vi "VGCServer.vi"() -> ()   [LabVIEW 2024]
doc: "Main control program for Aberystwyth Thermal Vacuum system"
uses:
  <vilib>/platform/TimedLoop/XDataNode/XDataNode.xnode
  Program Files/National Instruments/LabVIEW 2024/instr.lib/PL Inficon VGC/PL Inficon VGC.lvclass
  <vilib>/Platform/TimedLoop/XDataNode/nitl_modes.ctl
  <vilib>/Platform/TimedLoop/XDataNode/XDNodeRunTimeDep.lvlib
  <vilib>/Platform/TimedLoop/XDataNode/wakeup.ctl
  <vilib>/Platform/TimedLoop/XDataNode/timing_clust.ctl
  controls/VGCState.ctl
  controls/Vac Graph Config.ctl
panel:
  in  "Save Settings on exit":bool=TRUE
  out "stopping":bool=TRUE
  in  "Exit":bool
  in  "Main Tabs":enum32{"Setup", "Operating", "ExportData"}(tab)
  out "Application:Kind":T1(ring)
  out "App Version":string
  out "device information":T2={"type"="VGC503", "model number"="398-483", "serial number"="7433", "firmware version"="1.07", "hardware version"="1.0"}
  out "Event log":string
  in  "Backing SP":T3={"mode"=2, "thresholds"={"lower"=1.0, "upper"=5.0}, "on"=TRUE} {"thresholds"."upper" format="%#_5g"; "thresholds"."lower" format="%#_5g"; "mode" items=["off", "on", "channel 1", "channel 2", "channel 3"]}
  in  "Chamber SP":T3={"mode"=3, "thresholds"={"lower"=0.0001, "upper"=0.0005}, "on"=TRUE} {"thresholds"."upper" format="%#_5e"; "thresholds"."lower" format="%#_5g"; "mode" items=["off", "on", "channel 1", "channel 2", "channel 3"]}
  in  "LogFile":path=path "C:/Users/Public/Documents/TVC Logs/platten1.xlsx"
  in  "Log Interval (s)":dbl=5.0 min=0.1 max=100.0
  in  "Enable":bool
  out "Pressures":waveform(dbl)[](graph)
  out "Chamber Good":bool=TRUE
  out "Backing Good":bool=TRUE
  in  "Vacuum Graph config":T4={"Log/Lin"=TRUE, "Show Backing"=TRUE, "Show Chamber"=TRUE}
  in  "Clear Vacuum Chart":bool
  out "Status Bar":string="Application exit."
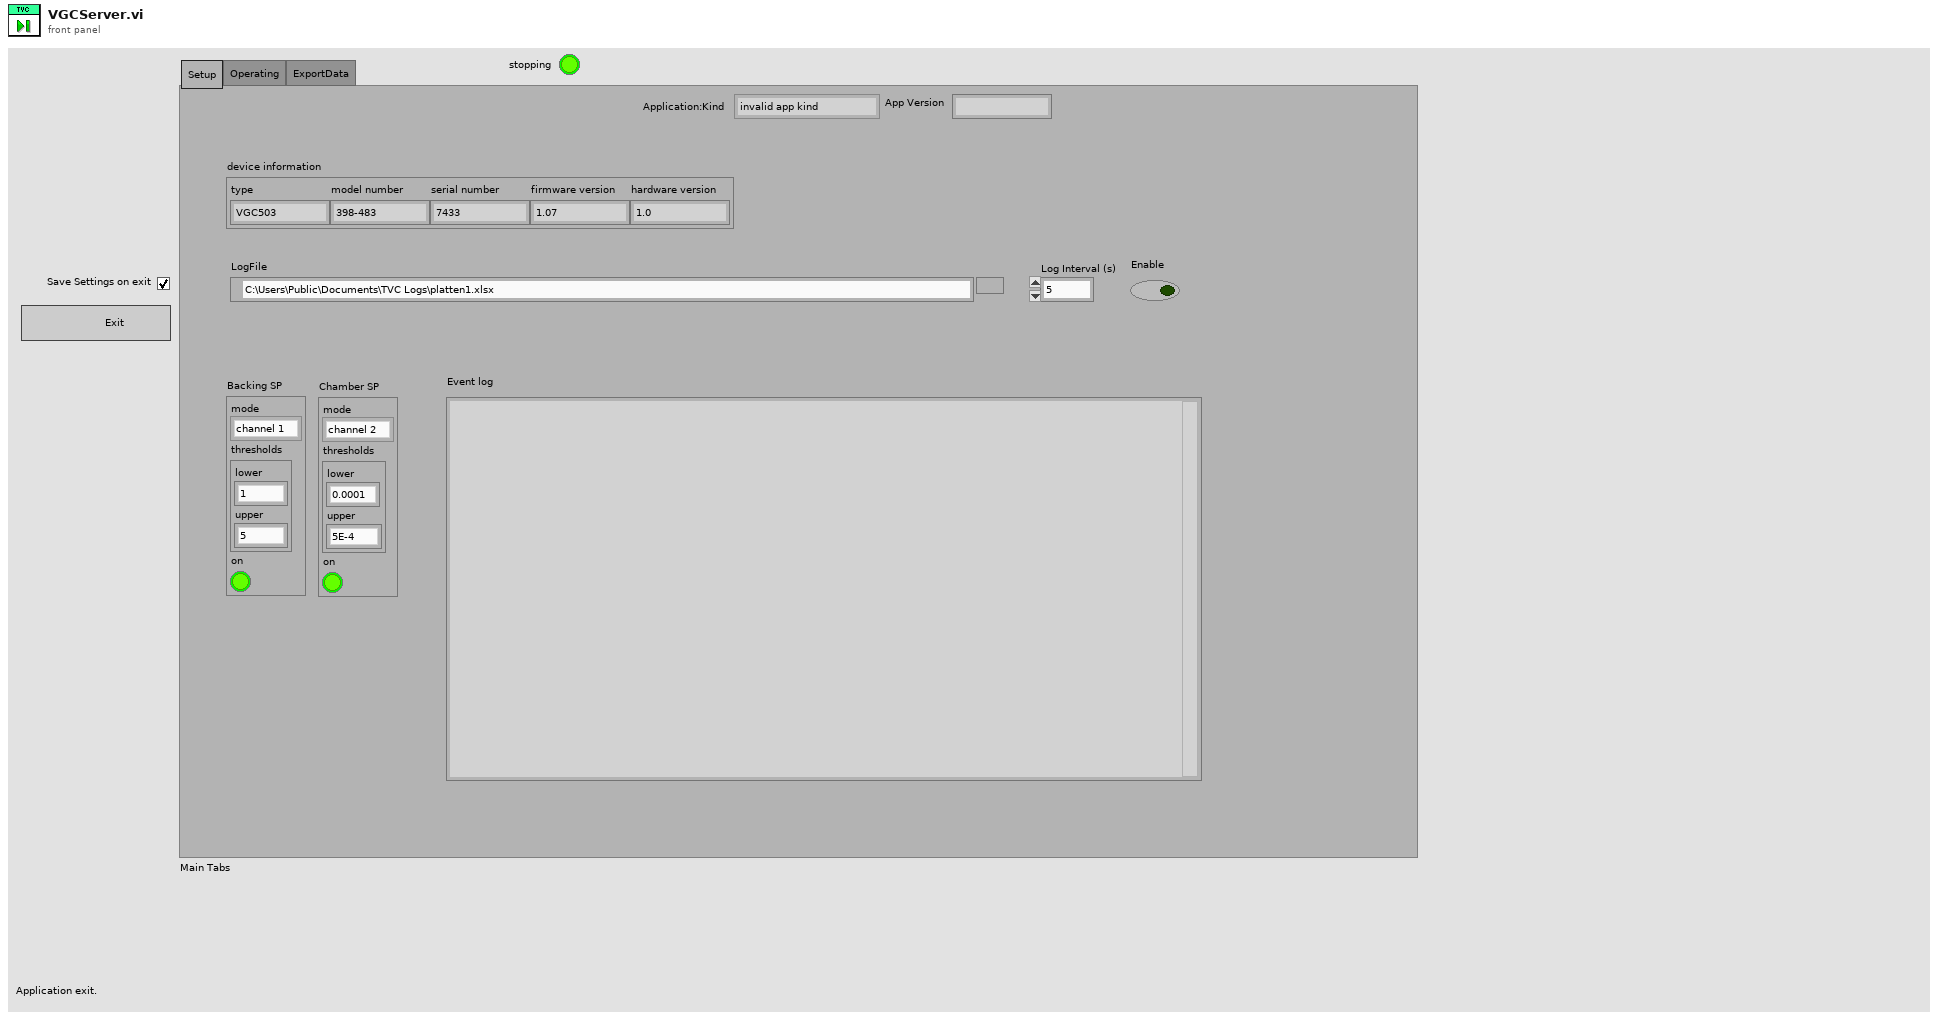
[diagram p1: front panel]
types:
  T1 = enum32{"invalid app kind", "Development System", "Run Time System", "Student Edition", "Embedded LabVIEW", "Evaluation", "Custom"}
  T2 = cluster{"type":string, "model number":string, "serial number":string, "firmware version":string, "hardware version":string}
  T3 = cluster{"mode":u16, "thresholds":cluster{"lower":dbl, "upper":dbl}, "on":bool}
  T4 = typedef "Vac Graph Config.ctl" = cluster{"Log/Lin":bool, "Show Backing":bool, "Show Chamber":bool}
  T5 = typedef "VGCState.ctl" = enum16{"Initialize", "InitHardware", "Wait for Event", "ShutDownHardware", "Exit"}
  T6 = typedef "VGCData.ctl" = cluster{"UI References":T7, "Vacuum Graph config":T4, "VGC50":T8}
  T7 = typedef "UI References.ctl" = cluster{"Exit Ref":refnum<vi>, "Save Ref":refnum<vi>, "Export Ref":refnum<vi>, "Acquire Ref":refnum<vi>, "Configure Ref":refnum<vi>, "Graph Ref":refnum<vi>, "Analyze Ref":refnum<vi>, "Status Ref":refnum<vi>, "Snapshot Ref":refnum<vi>, "Start Ref":refnum<vi>}
  T8 = typedef "VGC50.ctl" = cluster{"serial settings":cluster{"port":refnum<visa-resource-name>, "baud rate":u32}, "device information":cluster{"type":string, "model number":string, "serial number":string, "firmware version":string, "hardware version":string}, "VGC":refnum<class "PL Inficon VGC.lvclass">, "Backing SP":cluster{"mode":u16, "thresholds":cluster{"lower":dbl, "upper":dbl}, "on":bool}, "Chamber SP":cluster{"mode":u16, "thresholds":cluster{"lower":dbl, "upper":dbl}, "on":bool}}
  T9 = typedef "XDNodeRunTimeDep.lvlib/timing_clust.ctl" = cluster{"Expected End [f-1]":u64, "Actual End [f-1]":u64, "Finished Late? [f-1]":bool, "Expected End [i-1]":u64, "Actual End [i-1]":u64, "Finished Late? [i-1]":bool, "Expected Start [i]":u64, "Actual Start [i]":u64, "Expected Start [f]":u64, "Actual Start [f]":u64, "Source Name":string, "Structure Name":string, "Period":i64, "Deadline":i64, "Offset":i64, "Start":i64, "Priority":i32, "Timeout":i32, "Mode":T10, "Wakeup Reason":T11, "Error":errorcluster, "Source Type":string, "Secondary Source Type":string, "Global End Time":u64, "Global Start Time":u64, "Frame Duration":u64, "Iteration Duration":u64, "Assigned CPU":i32, "I/O Scan Engine Mode":u32}
  T10 = typedef "XDNodeRunTimeDep.lvlib/nitl_modes.ctl" = enum32{"No Change", "Process missed periods, maintain original phase", "Discard missed periods, maintain original phase", "Process missed periods, ignore original phase", "Discard missed periods, ignore original phase"}
  T11 = typedef "XDNodeRunTimeDep.lvlib/wakeup.ctl" = enum32{"Normal", "Aborted", "Asynchronous wakeup", "Timing source error", "Timed loop error", "Timeout"}
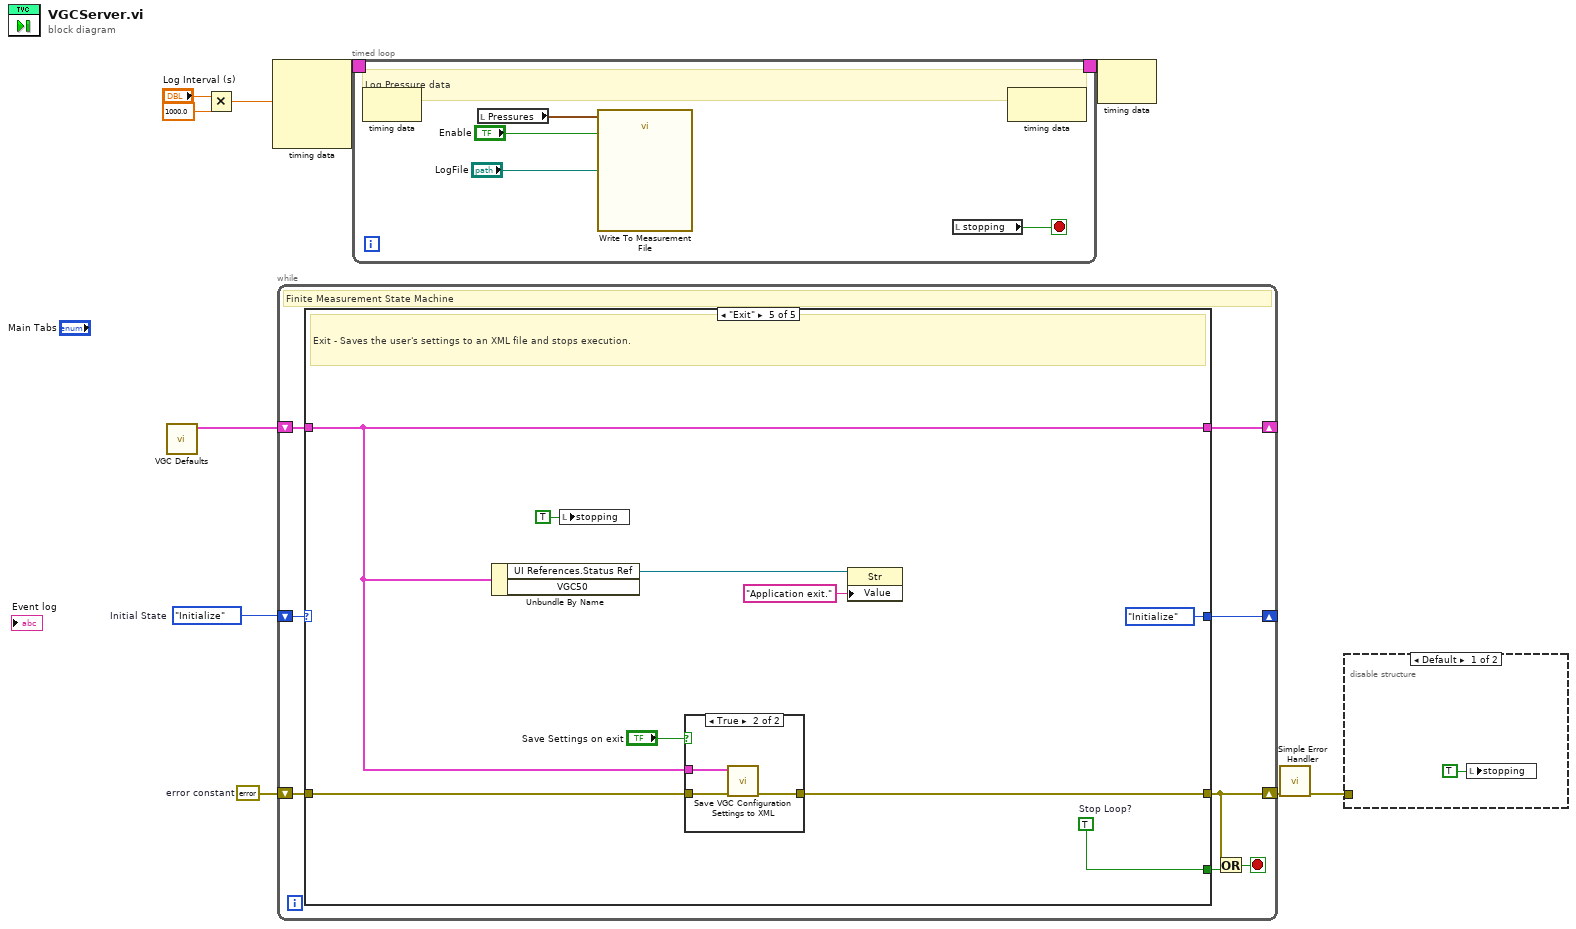
[diagram p0: block diagram]
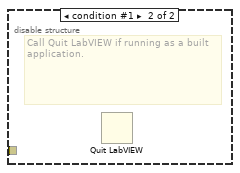
[diagram p2: hidden frame]
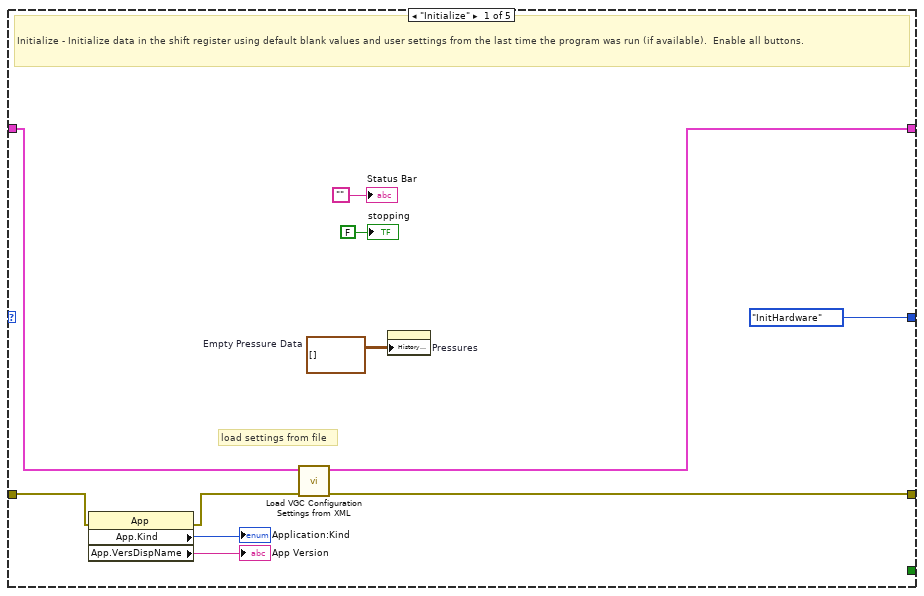
[diagram p3: hidden frame]
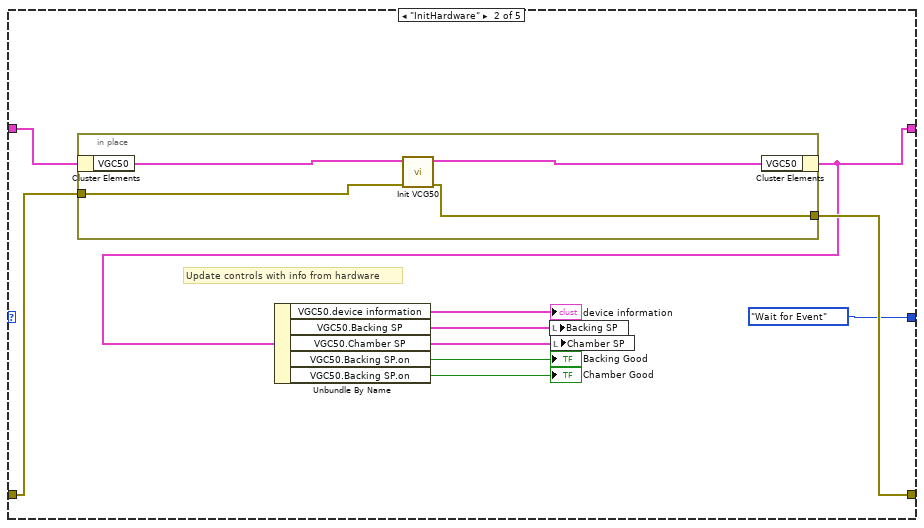
[diagram p4: hidden frame]
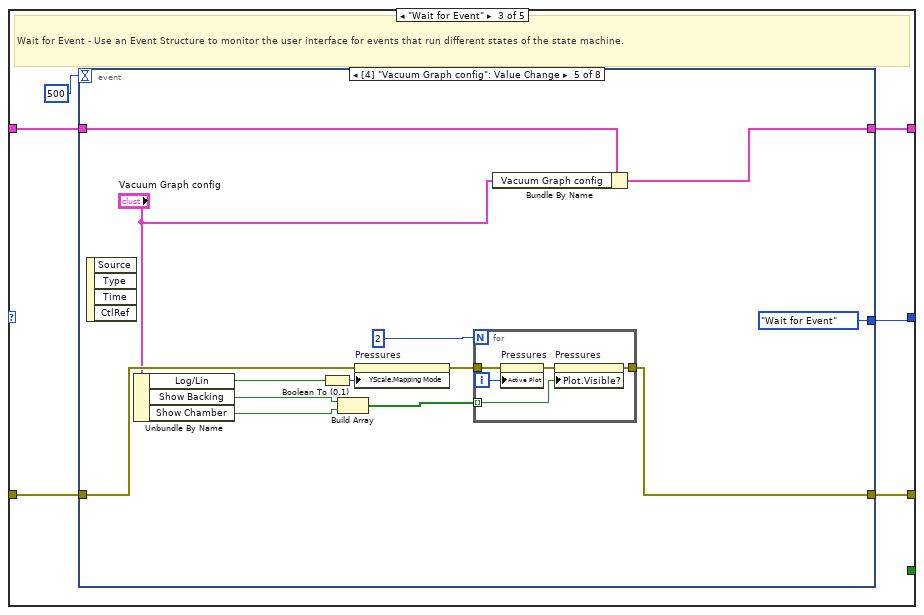
[diagram p5: hidden frame]
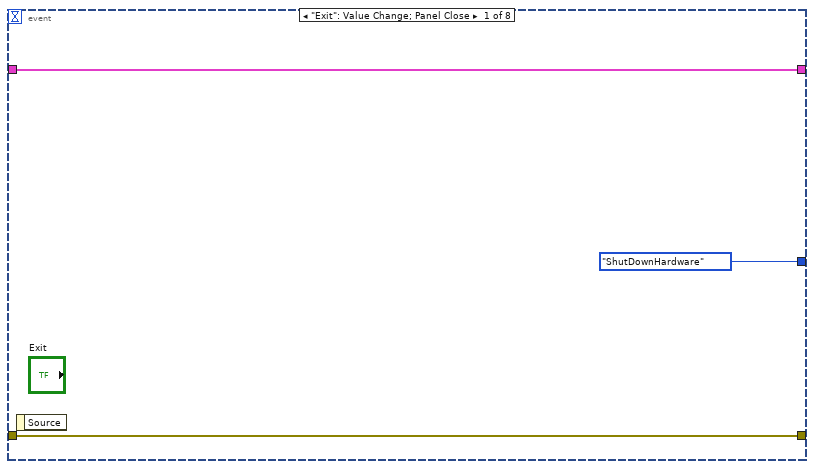
[diagram p6: hidden frame]
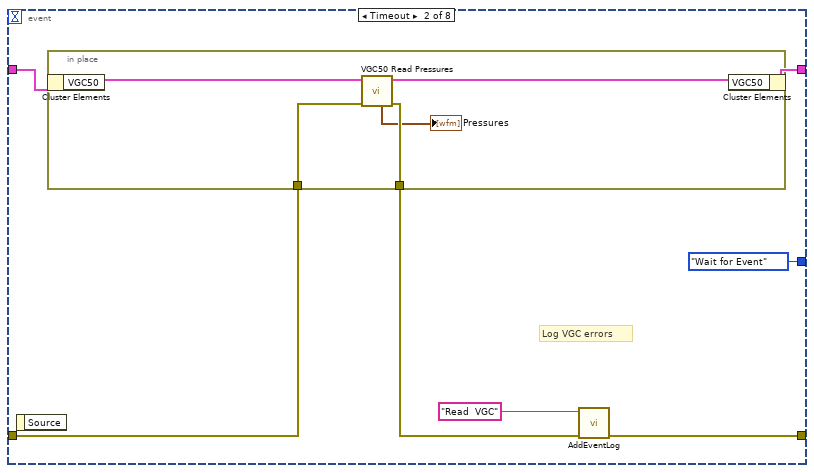
[diagram p7: hidden frame]
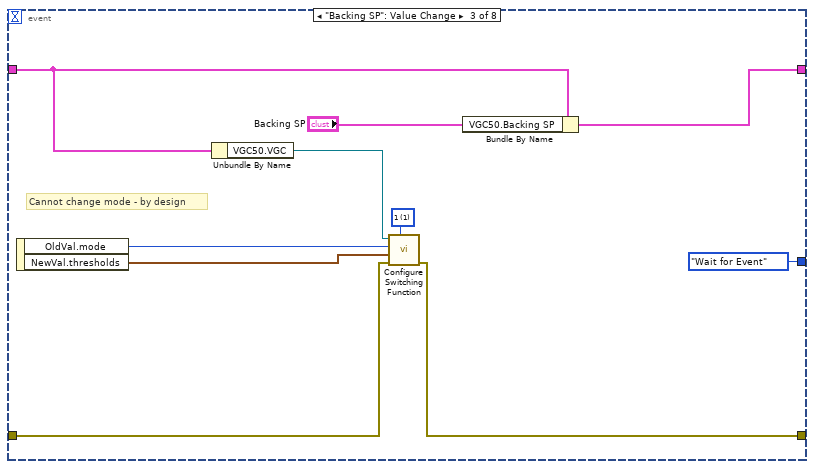
[diagram p8: hidden frame]
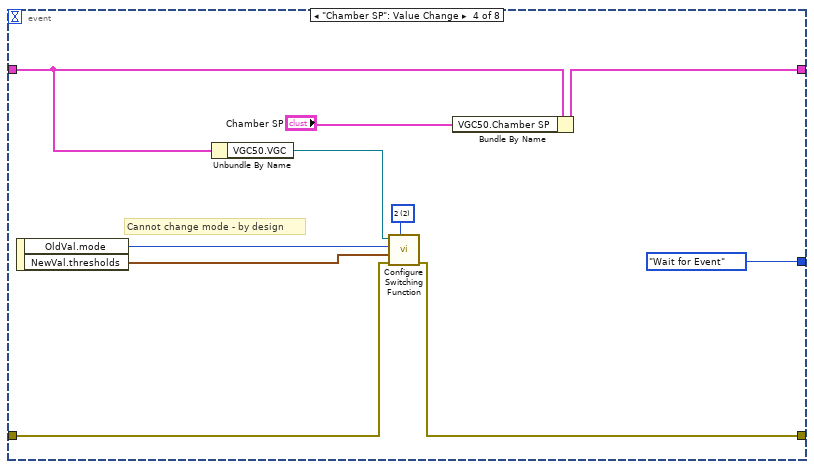
[diagram p9: hidden frame]
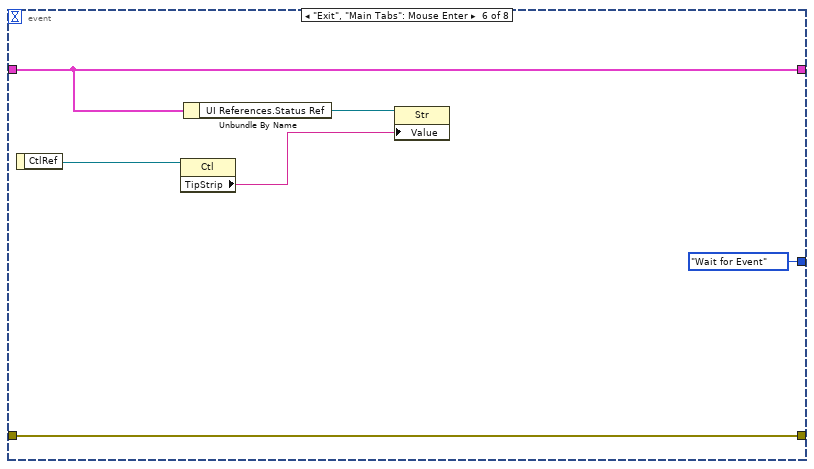
[diagram p10: hidden frame]
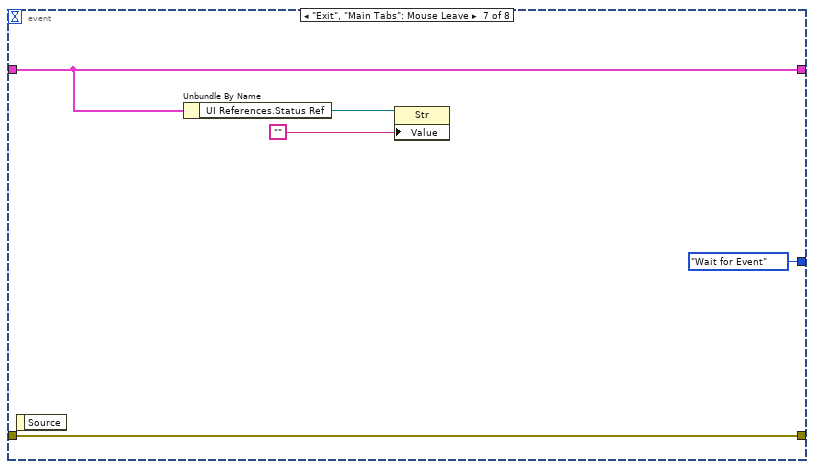
[diagram p11: hidden frame]
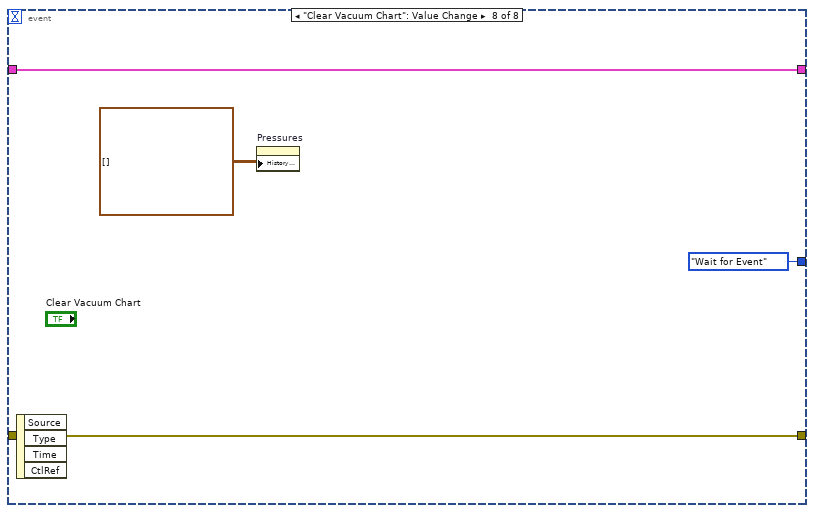
[diagram p12: hidden frame]
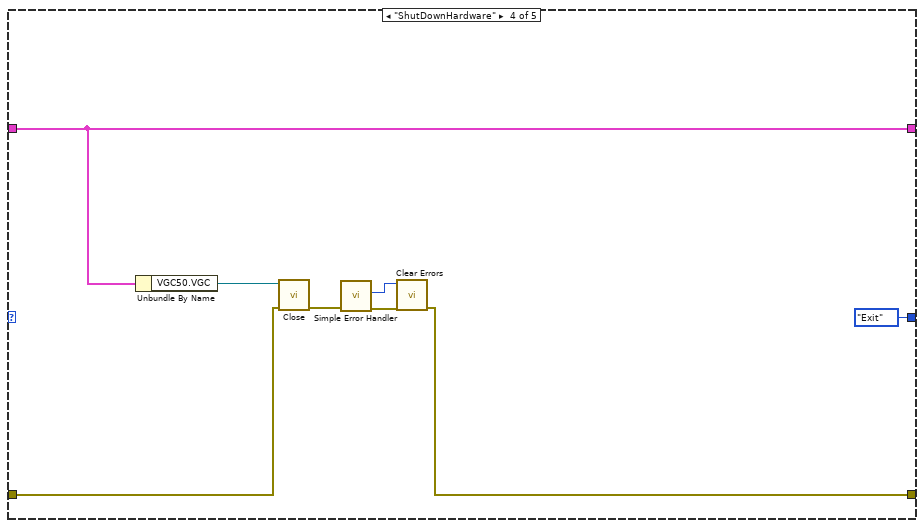
[diagram p13: hidden frame]
diagram:
  w9 = errorcluster {"status"=FALSE, "code"=0, "source"=""}  # error constant
  w10 = VGCState."Initialize"  # Initial State
  n1 = call "VGC Defaults.vi"() -> ("Data"=w6:T6)  [unwired: 11 in]
  n2 = Multiply(x="Log Interval (s)", y=1000.0) -> (x*y=w1:dbl)
  n3 = node-c288(w1) -> (w5:T9)  [unwired: 3 in]
  n4 = while {
    shift-right: [w11] -> _
    shift-left: w10 -> [w18]
    shift-right: [w16] -> _
    shift-left: w6 -> [w17]
    shift-right: [w12] -> w8
    shift-left: w9 -> [w15]
    stop <- w13 stop-if-true
    # "Finite Measurement State Machine"
    n5 = case shown="\"Exit\"" w18 {
      tunnel: [_ _ _ _ w134] -> w14
      tunnel: w17 -> [w20 w32 w49 w119 w126]
      tunnel: [w19 w31 w48 w119 w126] -> w16
      tunnel: w15 -> [w25 w39 w47 w121 w131]
      tunnel: [w29 w38 w46 w125 w130] -> w12
      tunnel: [VGCState."InitHardware" ("Initial State") VGCState."Wait for Event" ("Initial State") w44 VGCState."Exit" ("Initial State") VGCState."Initialize" ("Initial State")] -> w11
      frame "Initialize" {
        w22 = waveform(dbl)[][] []  # Empty Pressure Data
        # "load settings from file"
        # "Initialize - Initialize data in the shift register using default blank values and user settings from the last time the program was run (if available).  Enable all buttons."
        n6 = property class="App"(error in=w25) -> (error out=w26:errorcluster, "App.Kind"=→"Application:Kind":T1, "App.VersDispName"=→"App Version":string)  [unwired: 1 in, 1 out]
        n7 = call "Load VGC Configuration Settings from XML.vi"("error in (no error)"=w26, "Data"=w20) -> ("error out"=w29:errorcluster, "User Specified Out"=w19:T6)  [unwired: 8 in]
        n8 = property on="Pressures" class="WFChart (strict)"("History Data"=w22) -> ()  [unwired: 2 in, 2 out]
        "Status Bar" <- "" ("Status Bar")
        "stopping" <- FALSE ("stopping")
      }
      frame "InitHardware" {
        # "Update controls with info from hardware"
        n9 = in-place {
          in-place-border: w39 -> [w41]
          in-place-border: [w40] -> w38
          n10 = in-place-cluster #1(w32) -> ("VGC50"=w43:T8)
          n11 = call "Init VCG50.vi"("error in (no error)"=w41, "VGC50 In"=w43) -> ("error out"=w40:errorcluster, "VGC50 Out"=w42:T8)  [unwired: 8 in]
          n12 = in-place-cluster #1("VGC50"=w42) -> (w31:T6)
        }
        n13 = Unbundle By Name(w31) -> ("VGC50.device information"=→"device information":T2, "VGC50.Backing SP"=w36:T3, "VGC50.Chamber SP"=w35:T3, "VGC50.Backing SP.on"=→"Backing Good":bool, "VGC50.Backing SP.on"=→"Chamber Good":bool)
        n14 = local write "Backing SP"(w36) -> ()
        n15 = local write "Chamber SP"(w35) -> ()
      }
      frame "Wait for Event" {
        # "Wait for Event - Use an Event Structure to monitor the user interface for events that run different states of the state machine."
        n16 = event shown="[4] \"Vacuum Graph config\": Value Change" {
          selector: _ -> [_ _ _ _ _ _ _ _]
          dyn-events: _ -> [_ _ _ _ _ _ _ _]
          timeout: 500 -> [_ _ _ _ _ _ _ _]
          tunnel: w49 -> [w52 w57 w74 w84 w96 w106 w112 w116]
          tunnel: [w52 w56 w73 w83 w95 w106 w112 w116] -> w48
          tunnel: w47 -> [w51 w55 w71 w82 w88 w108 w113 w117]
          tunnel: [w51 w59 w67 w77 w87 w108 w113 w117] -> w46
          tunnel: [VGCState."ShutDownHardware" ("Initial State") VGCState."Wait for Event" ("Initial State") VGCState."Wait for Event" ("Initial State") VGCState."Wait for Event" ("Initial State") VGCState."Wait for Event" ("Initial State") VGCState."Wait for Event" ("Initial State") VGCState."Wait for Event" ("Initial State") VGCState."Wait for Event" ("Initial State")] -> w44
          event "Exit": Value Change; Panel Close {
            n17 = event-data() -> ()  [unwired: 1 in, 1 out]
          }
          event Timeout {
            # "Log VGC errors"
            n18 = event-data() -> ()  [unwired: 1 in, 1 out]
            n19 = in-place {
              in-place-border: w55 -> [w64]
              in-place-border: [w63] -> w54
              n20 = in-place-cluster #2(w57) -> ("VGC50"=w61:T8)
              n21 = call "VGC50 Read Pressures.vi"("error in (no error)"=w64, "VGC50 In"=w61) -> ("error out"=w63:errorcluster, "VGC50 Out"=w62:T8, "Waveform Chart"=→"Pressures":waveform(dbl)[])  [unwired: 5 in, 2 out]
              n22 = in-place-cluster #2("VGC50"=w62) -> (w56:T6)
            }
            n23 = call "AddEventLog.vi"("error in (no error)"=w54, "Event"="Read  VGC") -> ("error out"=w59:errorcluster)  [unwired: 9 in]
          }
          event "Backing SP": Value Change {
            w68 = u16 1 items=["1"=1, "2"=2, "3"=3, "4"=4, "5"=5, "6"=6] ("function")
            # "Cannot change mode - by design"
            n24 = event-data() -> ("OldVal.mode"=w66:u16, "NewVal.thresholds"=w70:cluster{"lower":dbl, "upper":dbl})  [unwired: 1 in]
            n25 = Unbundle By Name(w74) -> ("VGC50.VGC"=w69:refnum<class "PL Inficon VGC.lvclass">)
            n26 = call "Configure Switching Function.vi"("function"=w68, "error in (no error)"=w71, "thresholds"=w70, "mode"=w66, "VGC in"=w69) -> ("error out"=w67:errorcluster)  [unwired: 3 in, 3 out]
            n27 = Bundle By Name(cluster=w74, "VGC50.Backing SP"="Backing SP") -> (w73:T6)
          }
          event "Chamber SP": Value Change {
            w78 = u16 2 items=["1"=1, "2"=2, "3"=3, "4"=4, "5"=5, "6"=6] ("function")
            # "Cannot change mode - by design"
            n28 = event-data() -> ("OldVal.mode"=w80:u16, "NewVal.thresholds"=w81:cluster{"lower":dbl, "upper":dbl})  [unwired: 1 in]
            n29 = Unbundle By Name(w84) -> ("VGC50.VGC"=w79:refnum<class "PL Inficon VGC.lvclass">)
            n30 = call "Configure Switching Function.vi"("function"=w78, "error in (no error)"=w82, "thresholds"=w81, "mode"=w80, "VGC in"=w79) -> ("error out"=w77:errorcluster)  [unwired: 3 in, 3 out]
            n31 = Bundle By Name(cluster=w84, "VGC50.Chamber SP"="Chamber SP") -> (w83:T6)
          }
          event Value Change {
            n32 = event-data() -> ()  [unwired: 1 in, 4 out]
            n33 = Unbundle By Name("Vacuum Graph config") -> ("Log/Lin"=w94:bool, "Show Backing"=w92:bool, "Show Chamber"=w91:bool)
            n34 = Boolean To (0,1)(Boolean=w94) -> (0, 1=w97:i16)
            n35 = Build Array(w92, w91) -> (w90:bool[])
            n36 = property on="Pressures" class="WFChart (strict)"(error in=w88, "YScale.Mapping Mode"=w97) -> (error out=w89:errorcluster)  [unwired: 1 in, 1 out]
            n37 = for {
              N: 2 -> [_]
              tunnel: w90 -> [w100] mode=indexing
              tunnel: w89 -> [w99]
              tunnel: [w98] -> w87
              i -> [w101]
              n38 = property on="Pressures" class="WFChart (strict)"(error in=w99, "Active Plot"=w101) -> (error out=w102:errorcluster)  [unwired: 1 in, 1 out]
              n39 = property on="Pressures" class="WFChart (strict)"(error in=w102, "Plot.Visible?"=w100) -> (error out=w98:errorcluster)  [unwired: 1 in, 1 out]
            }
            n40 = Bundle By Name(cluster=w96, "Vacuum Graph config"="Vacuum Graph config") -> (w95:T6)
          }
          event "Exit", "Main Tabs": Mouse Enter {
            n41 = event-data() -> ("CtlRef"=w107:refnum<vi>)  [unwired: 1 in]
            n42 = property class="Ctl"(reference=w107) -> ("TipStrip"=w104:string)  [unwired: 1 in, 2 out]
            n43 = Unbundle By Name(w106) -> ("UI References.Status Ref"=w105:refnum<vi>)
            n44 = property class="Str"(reference=w105, "Value"=w104) -> ()  [unwired: 1 in, 2 out]
          }
          event "Exit", "Main Tabs": Mouse Leave {
            n45 = event-data() -> ()  [unwired: 1 in, 1 out]
            n46 = Unbundle By Name(w112) -> ("UI References.Status Ref"=w111:refnum<vi>)
            n47 = property class="Str"(reference=w111, "Value"="") -> ()  [unwired: 1 in, 2 out]
          }
          event "Clear Vacuum Chart": Value Change {
            n48 = event-data() -> ()  [unwired: 1 in, 4 out]
            n49 = property on="Pressures" class="WFChart (strict)"("History Data"=waveform(dbl)[][] []) -> ()  [unwired: 2 in, 2 out]
          }
        }
      }
      frame "ShutDownHardware" {
        n50 = Unbundle By Name(w119) -> ("VGC50.VGC"=w118:refnum<class "PL Inficon VGC.lvclass">)
        n51 = call "Close.vi"("error in (no error)"=w121, "VGC in"=w118) -> ("error out"=w123:errorcluster)  [unwired: 9 in]
        n52 = call <vilib>:"Simple Error Handler.vi"("error in (no error)"=w123) -> ("code out"=w124:i32, "error out"=w122:errorcluster)  [unwired: 4 in, 3 out]
        n53 = call <vilib>:"Clear Errors.vi"("error in (no error)"=w122, "specific error code to clear (0: all)"=w124) -> ("error out"=w125:errorcluster)  [unwired: 4 in, 1 out]
      }
      frame "Exit" {
        w134 = TRUE  # Stop Loop?
        # "Exit - Saves the user's settings to an XML file and stops execution."
        n54 = Unbundle By Name(w126) -> ("UI References.Status Ref"=w132:refnum<vi>)  [unwired: 1 out]
        n55 = local write "stopping"(TRUE ("stopping")) -> ()
        n56 = case shown="True" "Save Settings on exit" {
          tunnel: w131 -> [w135 w138]
          tunnel: [w135 w137] -> w130
          tunnel: w126 -> [_ w136]
          frame False {
          }
          frame True {
            n57 = call "Save VGC Configuration Settings to XML.vi"("error in (no error)"=w138, "User Configuration"=w136) -> ("error out"=w137:errorcluster)  [unwired: 9 in]
          }
        }
        n58 = property class="Str"(reference=w132, "Value"="Application exit." ("Stopped")) -> ()  [unwired: 1 in, 2 out]
      }
    }
    n59 = Or(x=w12, y=w14) -> (x .or. y?=w13:bool)
  }
  n60 = timed-loop {
    timing: w5 -> [_]
    timing-out: [_] -> w4
    stop <- w141 stop-if-true
    # "Log Pressure data"
    n61 = node-c288() -> ()  [unwired: 1 in, 1 out]
    n62 = local read "Pressures"() -> (w139:waveform(dbl)[])
    n63 = call "Write To Measurement File"("Signals"=w139, "Enable"="Enable", "Filename"="LogFile") -> ()  [unwired: 14 in, 3 out]
    n64 = local read "stopping"() -> (w141:bool)
    n65 = node-c288() -> ()  [unwired: 1 in, 1 out]
  }
  n66 = node-c288(w4) -> ()  [unwired: 1 out]
  n67 = call <vilib>:"Simple Error Handler.vi"("error in (no error)"=w8) -> ("error out"=w7:errorcluster)  [unwired: 4 in, 4 out]
  n68 = disable-structure shown="Default" {
    disable-tunnel: w7 -> [_ _]
    frame condition #0 (active) {
      n69 = local write "stopping"(TRUE ("stopping")) -> ()
    }
    frame condition #1 {
      # "Call Quit LabVIEW if running as a built application."
      n70 = Quit LabVIEW() -> ()  [unwired: 1 in]
    }
  }
